vi "isInheritance.vi"(0 "reference":refnum<class "ClassRelationshipEdge.lvclass">, 5 "error in (no error)":errorcluster) -> (14 "reference out":refnum<class "ClassRelationshipEdge.lvclass">, 15 "isInheritance":bool, 16 "isCompAggregation":bool, 19 "error out":errorcluster)   [LabVIEW 2012, in "ClassRelationshipEdge.lvclass"]
doc: "Returns TRUE if Edge is a inheritance type"
uses:
  <resource>/Framework/Providers/Open_GDS/UML/ClassRelationshipEdge_class/ClassRelationshipEdge.lvclass
  <resource>/Framework/Providers/Open_GDS/UML/ArrowHead_class/ArrowHead.lvclass
  <resource>/Framework/Providers/Open_GDS/UML/LineStyle_class/LineStyle.lvclass
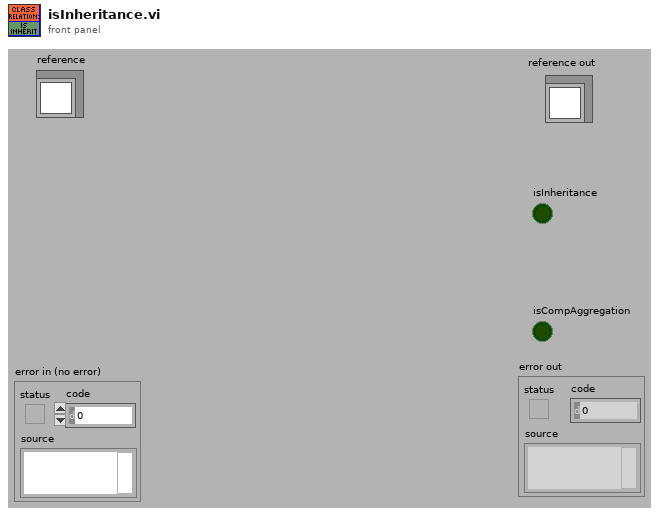
[diagram p1: front panel]
types:
  T1 = typedef "ClassRelationshipEdge.lvclass/ObjectAttributes.ctl" = cluster{"Base class":T2, "bentStyleRef":refnum<class "BentStyle.lvclass">, "startConnectionOffset":cluster{"x":i32, "y":i32}, "endConnectionOffset":cluster{"x":i32, "y":i32}, "MidLineOffset":cluster{"x":i32, "y":i32}, "DepClass":T6}
  T2 = typedef "SegmentedLineEdge.lvclass/ObjectAttributes.ctl" = cluster{"Base class":T3, "lineStyle":refnum<class "LineStyle.lvclass">, "startArrowHead":refnum<class "ArrowHead.lvclass">, "endArrowHead":refnum<class "ArrowHead.lvclass">, "startLabel":string, "midLabel":string, "endLabel":string, "MidLabelOffset":T5, "SplitWire":bool}
  T3 = typedef "GeneralPathEdge.lvclass/ObjectAttributes.ctl" = cluster{"Base class":T4}
  T4 = typedef "AbstractEdge.lvclass/ObjectAttributes.ctl" = cluster{"start":refnum<class "AbstractNode.lvclass">, "end":refnum<class "AbstractNode.lvclass">}
  T5 = typedef "Point Point2D.ctl" = cluster{"x":dbl, "y":dbl}
  T6 = typedef "ReversedEngineering_ViDependencyDetailsType.ctl" = cluster{"ThisVIs/Ctls":path[], "Dependent_VIs/Ctls":path[]}
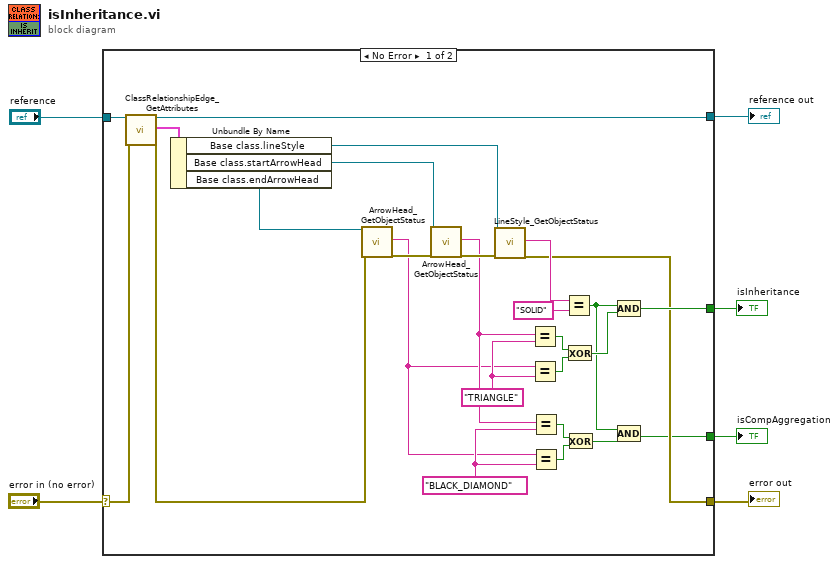
[diagram p0: block diagram]
diagram:
  n1 = case shown="No Error" "error in (no error)" {
    selector: "error in (no error)" -> [w32 w33]
    tunnel: "reference" -> [w31 w34]
    tunnel: [w18 w33] -> w4
    tunnel: [w29 w34] -> w3
    tunnel: [w19 _] -> w2
    tunnel: [w7 _] -> w1
    frame No Error {
      w12 = "BLACK_DIAMOND" ("y")
      w25 = "TRIANGLE" ("y")
      n2 = call <resource>:"ClassRelationshipEdge_GetAttributes.vi"("reference in"=w31, "error in (no error)"=w32) -> ("reference out"=w29:refnum<class "ClassRelationshipEdge.lvclass">, "Attributes"=w30:T1, "error out"=w27:errorcluster)  [unwired: 15 out]
      n3 = Unbundle By Name(w30) -> ("Base class.lineStyle"=w22:refnum<class "LineStyle.lvclass">, "Base class.startArrowHead"=w26:refnum<class "ArrowHead.lvclass">, "Base class.endArrowHead"=w28:refnum<class "ArrowHead.lvclass">)
      n4 = call <resource>:"ArrowHead_GetObjectStatus.vi"("reference in"=w28, "error in (no error)"=w27) -> ("Object name"=w10:string, "error out"=w24:errorcluster)  [unwired: 16 out]
      n5 = call <resource>:"ArrowHead_GetObjectStatus.vi"("reference in"=w26, "error in (no error)"=w24) -> ("Object name"=w11:string, "error out"=w23:errorcluster)  [unwired: 16 out]
      n6 = call <resource>:"LineStyle_GetObjectStatus.vi"("reference"=w22, "error in (no error)"=w23) -> ("Type(String)"=w21:string, "error out"=w18:errorcluster)  [unwired: 15 in, 1 out]
      n7 = Equal?(x=w11, y=w25) -> (x = y?=w17:bool)
      n8 = Equal?(x=w10, y=w25) -> (x = y?=w16:bool)
      n9 = Equal?(x=w11, y=w12) -> (x = y?=w13:bool)
      n10 = Equal?(x=w10, y=w12) -> (x = y?=w14:bool)
      n11 = Equal?(x=w21, y="SOLID") -> (x = y?=w8:bool)
      n12 = Exclusive Or(1:w16, 2:w17) -> (0:w15:bool)
      n13 = Exclusive Or(1:w14, 2:w13) -> (0:w9:bool)
      n14 = Compound Arithmetic op=AND(w8, w15) -> (w19:bool)
      n15 = Compound Arithmetic op=AND(w8, w9) -> (w7:bool)
    }
    frame Error {
    }
  }
  "reference out" <- w3
  "error out" <- w4
  "isInheritance" <- w2
  "isCompAggregation" <- w1
